vi "Save Data.vi"(8 "error in (no error)":errorcluster, 11 "Data":waveform(dbl)[](array[waveform])) -> (0 "error out":errorcluster)   [LabVIEW 2022 SP3]
doc: "Saves data to disk in the TDMS file format."
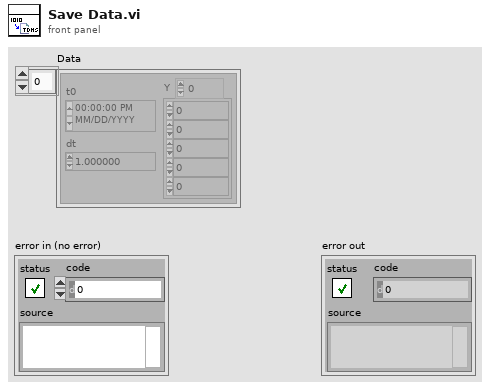
[diagram p1: front panel]
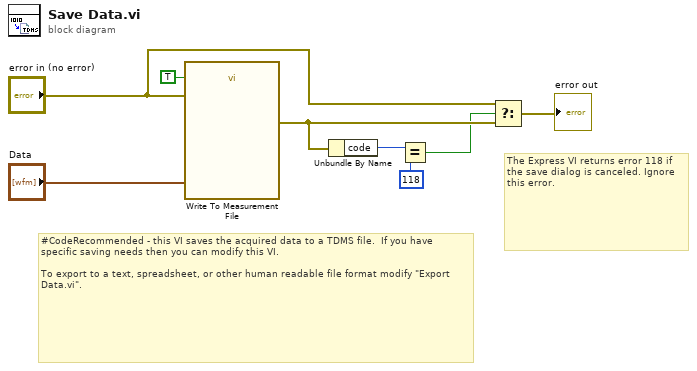
[diagram p0: block diagram]
diagram:
  # "The Express VI returns error 118 if the save dialog is canceled. Ignore this error."
  # "#CodeRecommended - this VI saves the acquired data to a TDMS file.  If you have specific saving needs then you can modify this VI.\n\nTo export to a text, spreadsheet, or other human readable file format modify \"Export Data.vi\"."
  n1 = call "Write To Measurement File"("Signals"="Data", "Reset"=TRUE, "error in (no error)"="error in (no error)") -> ("error out"=w5:errorcluster)  [unwired: 14 in, 2 out]
  n2 = Unbundle By Name(w5) -> ("code"=w3:i32)
  n3 = Equal?(x=w3, y=118) -> (x = y?=w2:bool)
  n4 = Select(t="error in (no error)", s=w2, f=w5) -> (s? t:f=→"error out":errorcluster)
